vi "changeHardpointStates.vi"(0 "Model in":refnum<class "Model.lvclass">, 5 "Mode":u16, 7 "WaitForTrigger":bool, 9 "TriggerIRQ":bool, 11 "error in (no error)":errorcluster) -> (4 "Model out":refnum<class "Model.lvclass">, 15 "error out":errorcluster)   [LabVIEW 2016, in "Model.lvclass"]
uses:
  Model.lvclass
  Model.lvclass/Model.ctl
  ILCCommunications/ILCCommunications.lvclass/ILCCommunications.ctl
  Common_RT_ILC/ILC/ILC.lvclass/ILC.ctl
  Common_RT_HPILC/HPILC/HPILC.lvclass
  D:/Code/ts_M1M3Support/Common_RT_ILC/ILC/ILC.lvclass
  ILCCommunications/ILCCommunications.lvclass
  Common_RT_ILC/ILC/ILC.lvclass
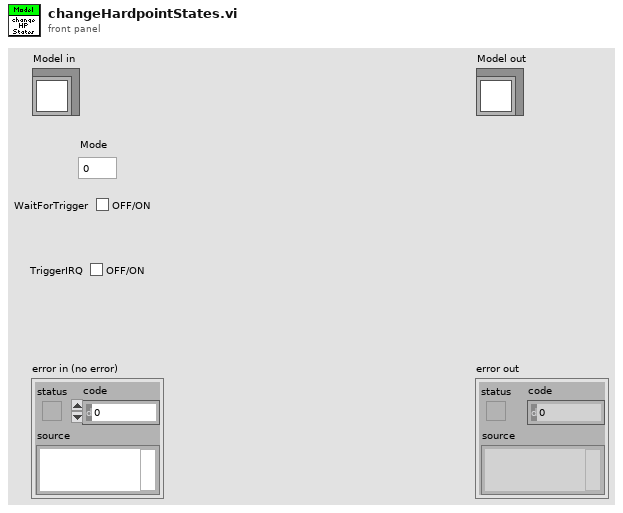
[diagram p1: front panel]
types:
  T1 = typedef "RTILC.lvlib/ILCData.ctl" = cluster{"Constants":T2, "Command":T3, "Telemetry":T5, "Responses":T6, "Timings":T8}
  T2 = typedef "RTILC.lvlib/ILCConstants.ctl" = cluster{"Subnet":u8, "Address":u8}
  T3 = typedef "RTILC.lvlib/ILCCommand.ctl" = cluster{"ILCMode":u16, "TemporaryAddress":u8, "ADCScanRate":T4, "ADCChannel":u8, "ADCOffset":sgl, "ADCSensitivity":sgl}
  T4 = typedef "RTILC.lvlib/ILCScanRates.ctl" = u8
  T5 = typedef "RTILC.lvlib/ILCTelemetry.ctl" = cluster{"UniqueID":u64, "FirmwareType":u8, "NetworkNodeType":u8, "ILCOption":u8, "NetworkNodeOption":u8, "MajorRevision":u8, "MinorRevision":u8, "FirmwareName":string, "ILCMode":u16, "MajorFault":bool, "MinorFault":bool, "FaultOverride":bool, "MainCalibrationError":bool, "BackupCalibrationError":bool, "UniqueIDCRCMismatch":bool, "AppTypeNodeTypeMismatch":bool, "AppMissing":bool, "AppCRCMismatch":bool, "TEDSNotFound":bool, "TEDS1Mismatch":bool, "TEDS2Mismatch":bool, "WatchdogResetDetected":bool, "BrownoutDetected":bool, "EventTrapResetDetected":bool, "MotorPowerFault":bool, "SSRPowerFault":bool, "AuxPowerFault":bool, "SMCPowerFault":bool, "TemporaryAddress":u8, "ADCScanRate":T4, "DAC1":u16, "DAC2":u16, "DAC3":u16, "DAC4":u16, "MainADCCalibrationK":sgl[], "MainSensorOffset":sgl[], "MainSensorSensitivity":sgl[], "BackupADCCalibrationK":sgl[], "BackupSensorOffset":sgl[], "BackupSensorSensitivity":sgl[]}
  T6 = typedef "RTILC.lvlib/ILCResponses.ctl" = cluster{"ReportServerID":T7, "ReportServerStatus":T7, "ILCMode":T7, "SetTemporaryAddress":T7, "Reset":T7, "ADCScanRate":T7, "ADCOffsetSensitivity":T7, "ReadDAC":T7, "ReadCalibration":T7}
  T7 = typedef "RTModbus.lvlib/ExceptionCodes.ctl" = u16
  T8 = typedef "RTILC.lvlib/ILCTimings.ctl" = cluster{"ADCOffsetSensitivity":u32, "ADCScanRate":u32, "ILCMode":u32, "ReadCalibration":u32, "ReportServerID":u32, "ReportServerStatus":u32, "Reset":u32, "SetTemporaryAddress":u32}
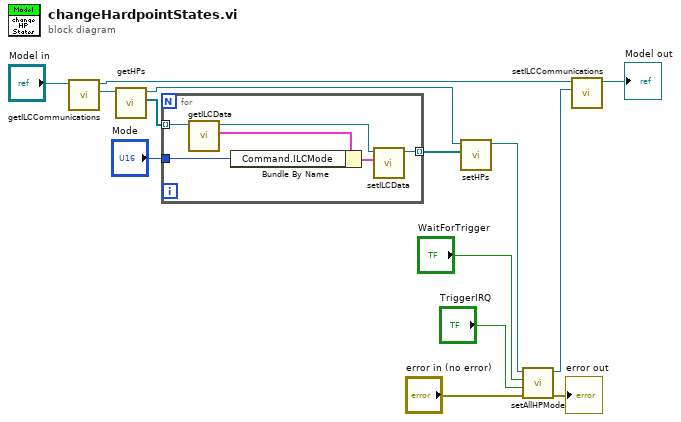
[diagram p0: block diagram]
diagram:
  n1 = call "getILCCommunications.vi"("Model in"="Model in") -> ("ILCCommunications"=w13:refnum<class "ILCCommunications.lvclass">, "Model out"=w2:refnum<class "Model.lvclass">)  [unwired: 9 in]
  n2 = call "getHPs.vi"("ILCCommunications in"=w13) -> ("HPs"=w5:refnum<class "HPILC.lvclass">[], "ILCCommunications out"=w6:refnum<class "ILCCommunications.lvclass">)  [unwired: 9 in]
  n3 = for {
    tunnel: w5 -> [w20] mode=indexing
    tunnel: [w18] -> w4 mode=indexing
    tunnel: "Mode" -> [w15]
    n4 = call "getILCData.vi"("ILC in"=w20) -> ("ILCData"=w17:T1, "ILC out"=w19:refnum<class "HPILC.lvclass">)  [unwired: 9 in]
    n5 = Bundle By Name(cluster=w17, "Command.ILCMode"=w15) -> (w16:T1)
    n6 = call "setILCData.vi"("ILCData"=w16, "ILC in"=w19) -> ("ILC out"=w18:refnum<class "HPILC.lvclass">)  [unwired: 9 in]
  }
  n7 = call "setHPs.vi"("HPs"=w4, "ILCCommunications in"=w6) -> ("ILCCommunications out"=w12:refnum<class "ILCCommunications.lvclass">)  [unwired: 9 in]
  n8 = call "setAllHPMode.vi"("error in (no error)"="error in (no error)", "TriggerIRQ"="TriggerIRQ", "WaitForTrigger"="WaitForTrigger", "ILCCommunications in"=w12) -> ("error out"=→"error out":errorcluster, "ILCCommunications out"=w7:refnum<class "ILCCommunications.lvclass">)  [unwired: 6 in]
  n9 = call "setILCCommunications.vi"("ILCCommunications"=w7, "Model in"=w2) -> ("Model out"=→"Model out":refnum<class "Model.lvclass">)  [unwired: 9 in]
